vi "Initialize Pickering.vi"(0 "Resource Name":string="PXI2::15::INSTR", 1 "Action":bool, 2 "Reset":bool, 3 "Error In (no error)":errorcluster) -> (10 "Error Out":errorcluster)   [LabVIEW 2015]
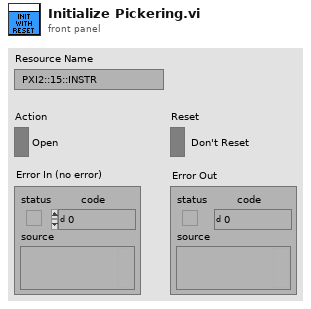
[diagram p1: front panel]
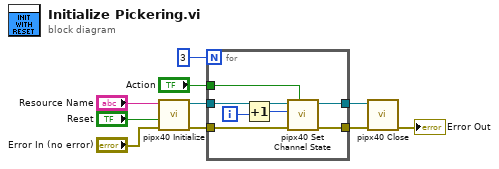
[diagram p0: block diagram]
diagram:
  n1 = call "pipx40 Initialize.vi"("error in (no error)"="Error In (no error)", "reset device"="Reset", "resource name"="Resource Name") -> ("error out"=w8:errorcluster, "instrument handle out"=w10:refnum<visa-resource-name>)  [unwired: 7 in]
  n2 = for {
    N: 3 -> [_]
    tunnel: w10 -> [w17]
    tunnel: w8 -> [w16]
    tunnel: "Action" -> [w15]
    tunnel: [w12] -> w2
    tunnel: [w11] -> w3
    i -> [w14]
    n3 = Increment(x=w14) -> (x+1=w13:i32)
    n4 = call "pipx40 Set Channel State.vi"("action"=w15, "error in (no error)"=w16, "subunit number"=w13, "instrument handle"=w17) -> ("error out"=w12:errorcluster, "instrument handle out"=w11:refnum<visa-resource-name>)  [unwired: 6 in]
  }
  n5 = call "pipx40 Close.vi"("error in (no error)"=w2, "instrument handle"=w3) -> ("error out"=→"Error Out":errorcluster)  [unwired: 9 in]
